vi "Image Display Save Image.vi"(6 "Mask Color (Transparent)":u32(colorbox)=16777216, 8 "error in (no error)":errorcluster, 9 "Saved Image File Format":T2, 10 "File Path in":path, 11 "Display Image Control Refnum":T1) -> (0 "Error Out":errorcluster, 2 "File Path out":path)   [LabVIEW 2021, in "Image.lvlib"]
uses:
  Image.lvlib
  Image Save File Format.ctl
  Image Control Refnum.ctl
  Selected Area in Object.ctl
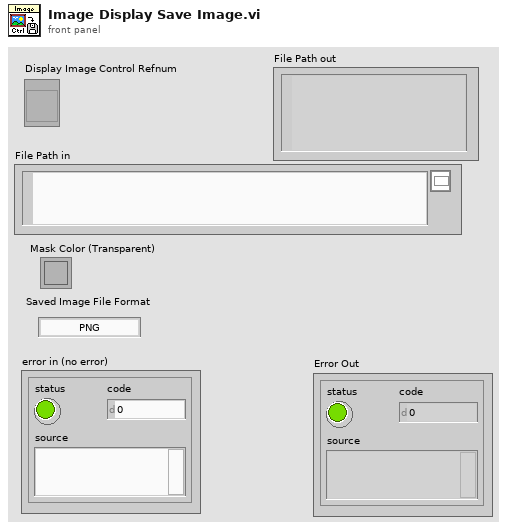
[diagram p1: front panel]
types:
  T1 = typedef "Image.lvlib/Image Control Refnum.ctl" = refnum<vi>
  T2 = typedef "Image.lvlib/Image Save File Format.ctl" = enum16{"PNG", "JPEG", "BMP"}
  T3 = typedef "Image.lvlib/Selected Area in Object.ctl" = cluster{"Selected Area Position Left":i32, "Selected Area Position Top":i32, "Selected Area Size Height":u32, "Selected Area Size Width":u32, "Object Position Left":i32, "Object Position Top":i32}
  T4 = typedef "imagedata.ctl" = cluster{"image type":i32, "image depth":i32, "image":u8[], "mask":u8[], "colors":u32[], "Rectangle":cluster{"left":i16, "top":i16, "right":i16, "bottom":i16}}
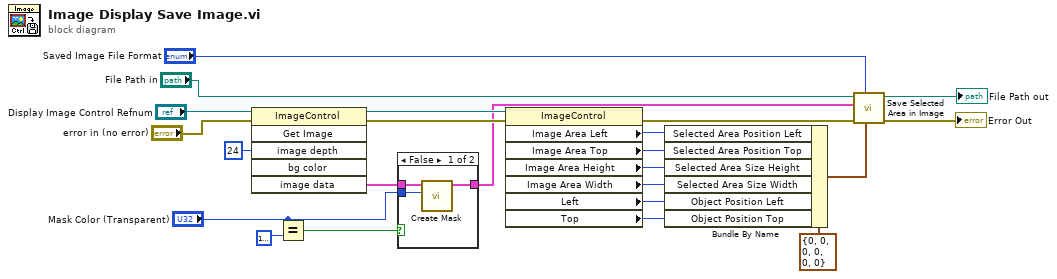
[diagram p0: block diagram]
diagram:
  n1 = invoke class="ImageControl" method="Get Image"(reference="Display Image Control Refnum", error in="error in (no error)", "image depth"=24 ("Image Depth")) -> (reference out=w20:T1, error out=w18:errorcluster, "image data"=w5:T4)  [unwired: 3 in, 3 out]
  n2 = Equal?(x="Mask Color (Transparent)", y=u32 16777216 ("Mask Color (Black)")) -> (x = y?=w2:bool)
  n3 = case shown="False" w2 {
    tunnel: w5 -> [w25 w27]
    tunnel: [w24 w27] -> w4
    tunnel: "Mask Color (Transparent)" -> [w26 _]
    frame False {
      n4 = call <vilib>:"Create Mask.vi"("Mask Color (Black)"=w26, "image data"=w25) -> ("image data"=w24:T4)  [unwired: 9 in]
    }
    frame True {
    }
  }
  n5 = property class="ImageControl"(reference=w20, error in=w18) -> (error out=w17:errorcluster, "Image Area Left"=w14:i32, "Image Area Top"=w13:i32, "Image Area Height"=w12:u32, "Image Area Width"=w11:u32, "Left"=w10:i32, "Top"=w9:i32)  [unwired: 1 out]
  n6 = Bundle By Name(cluster=T3 {"Selected Area Position Left"=0, "Selected Area Position Top"=0, "Selected Area Size Height"=0, "Selected Area Size Width"=0, "Object Position Left"=0, "Object Position Top"=0} ("output cluster"), "Selected Area Position Left"=w14, "Selected Area Position Top"=w13, "Selected Area Size Height"=w12, "Selected Area Size Width"=w11, "Object Position Left"=w10, "Object Position Top"=w9) -> (w7:T3)
  n7 = call "Save Selected Area in Image.vi"("Selected Area in Object"=w7, "Saved Image File Format"="Saved Image File Format", "error in (no error)"=w17, "Image Data"=w4, "File Path in"="File Path in") -> ("error out"=→"Error Out":errorcluster, "File Path out"=→"File Path out":path)  [unwired: 5 in]
